vi "getLN2Level.vi"(8 "error in (no error)":errorcluster, 11 "Instrument.Cryostat in":refnum<class "Instrument.Cryostat.lvclass">) -> (0 "error out":errorcluster, 2 "LN2 Level (%)":dbl, 3 "Instrument.Cryostat out":refnum<class "Instrument.Cryostat.lvclass">)   [LabVIEW 2019, in "Instrument.Cryostat.lvclass"]
uses:
  Instrument.Cryostat.lvclass
  C:/Users/patrick/Documents/GitHub/Instrument-Framework/lvsrc/Instrument/Instrument.lvclass
  Instrument/Instrument.lvclass/Instrument.ctl
  6256ba45-6158-46f1-bca1-f27db6896cf6.vi
  6256ba45-6158-46f1-bca1-f27db6896cf6.vi/a7f4cbe1-ceb0-4a1d-a837-22c43e128834.vi
  Instrument/API/Send and Receive.vi
  6256ba45-6158-46f1-bca1-f27db6896cf6.vi/b50c56e5-2be5-4fe8-90d4-5774baab1b1e.vi
  Instrument/Private/Get Client Type.vi
  6256ba45-6158-46f1-bca1-f27db6896cf6.vi/a7f4cbe1-ceb0-4a1d-a837-22c43e128834.vi/65b94138-0124-4a04-931c-0e88de16b5a4.vi
  6256ba45-6158-46f1-bca1-f27db6896cf6.vi/a7f4cbe1-ceb0-4a1d-a837-22c43e128834.vi/e6665fc2-246b-4a33-9a88-3097d89a11c8.vi
  6256ba45-6158-46f1-bca1-f27db6896cf6.vi/b50c56e5-2be5-4fe8-90d4-5774baab1b1e.vi/e93db6c8-b69d-4428-b841-44bc44a80f29.vi
  6256ba45-6158-46f1-bca1-f27db6896cf6.vi/b50c56e5-2be5-4fe8-90d4-5774baab1b1e.vi/0e365ba2-d04c-4076-82c5-04f9ead79f82.vi
  6256ba45-6158-46f1-bca1-f27db6896cf6.vi/b50c56e5-2be5-4fe8-90d4-5774baab1b1e.vi/e93db6c8-b69d-4428-b841-44bc44a80f29.vi/927b8a84-0505-49e8-921a-832ed2dabb50.vi
  6256ba45-6158-46f1-bca1-f27db6896cf6.vi/b50c56e5-2be5-4fe8-90d4-5774baab1b1e.vi/e93db6c8-b69d-4428-b841-44bc44a80f29.vi/9e239a84-7e7b-4ffc-9ef8-d9081babd39c.vi
  Instrument/Private/Get RC Connection Status.vi
  Instrument/API/Enum to String.vi
  <userlib>/LevyLab/RemoteControl/API/Send and Receive.vi
  <vilib>/Utility/Data Type/Get Type Information.vi
  <vilib>/JDP Science/JSONtext/JSON text to Variant.vi
  Instrument/API/Instrument.GetPublicEvents.vi
  <vilib>/JDP Science/JSONtext/Variant to JSON Text.vi
  <vilib>/National Instruments/GUID Generator/Guid Generator.vi
  Instrument/API/Instrument.sendMessageToProcess.vi
  Instrument/Private/Instrument.MessageFromProcess.EventStructure.vi
  <vilib>/JDP Science/JSONtext/LVClass Serializer/JSONtext LVClass Serializer.lvclass
  Instrument/Instrument.lvclass
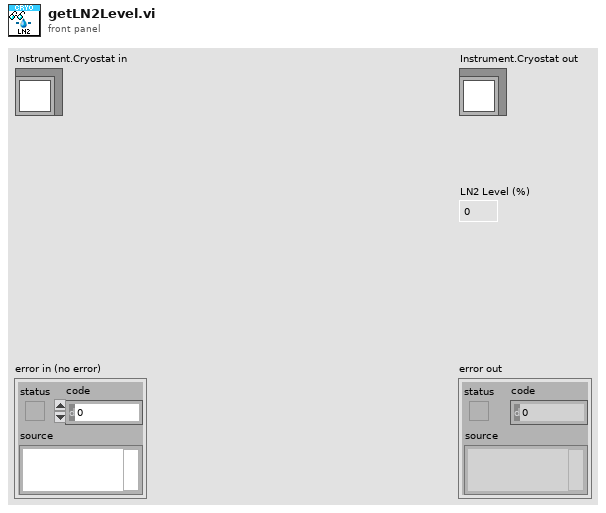
[diagram p1: front panel]
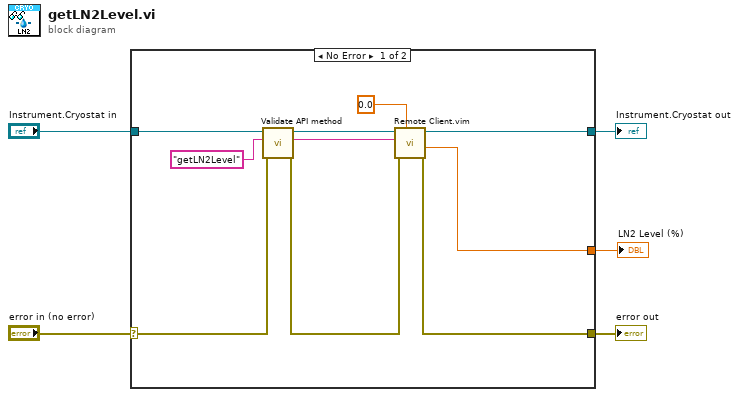
[diagram p0: block diagram]
diagram:
  n1 = case shown="No Error" "error in (no error)" {
    selector: "error in (no error)" -> [w6 w17]
    tunnel: [w14 w17] -> w4
    tunnel: [w13 w16] -> w2
    tunnel: "Instrument.Cryostat in" -> [w9 w16]
    tunnel: [w15 _] -> w1
    frame No Error {
      n2 = call "Validate API method.vi"("error in (no error)"=w6, "command in"="getLN2Level" ("error message (\"\")"), "Instrument in"=w9) -> ("error out"=w12:errorcluster, "command out"=w8:string, "Instrument out"=w7:refnum<class "Instrument.Cryostat.lvclass">)  [unwired: 6 in]
      n3 = call "Remote Client.vim"("Data Out type"=0.0, "error in (no error)"=w12, "method"=w8, "Instrument in"=w7) -> ("error out"=w14:errorcluster, "Data out"=w15:dbl, "Instrument out"=w13:refnum<class "Instrument.Cryostat.lvclass">)  [unwired: 4 in, 1 out]
    }
    frame Error {
    }
  }
  "error out" <- w4
  "Instrument.Cryostat out" <- w2
  "LN2 Level (%)" <- w1
